vi "ConfigureTarget.vi"(8 "error in (no error)":errorcluster, 10 "TargetRate":dbl, 11 "Target Reference in":refnum<k24>) -> (0 "error out":errorcluster, 3 "Target Reference out":refnum<k24>)   [LabVIEW 2015, in "VeriStandTestUtilities.lvlib"]
uses:
  VeriStandTestUtilities.lvlib
  NationalInstruments.VeriStand.SystemDefinitionAPI
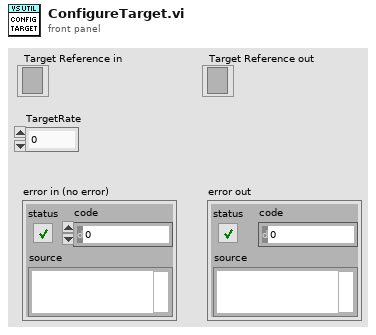
[diagram p1: front panel]
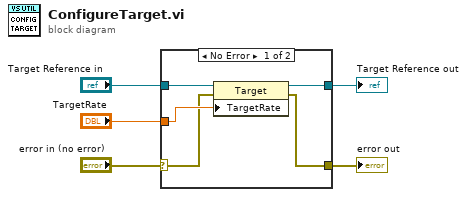
[diagram p0: block diagram]
diagram:
  n1 = case shown="No Error" "error in (no error)" {
    selector: "error in (no error)" -> [w6 w12]
    tunnel: [w10 w12] -> w5
    tunnel: [w9 w11] -> w4
    tunnel: "Target Reference in" -> [w8 w11]
    tunnel: "TargetRate" -> [w7 _]
    frame No Error {
      n2 = property class="Target"(reference=w8, error in=w6, "TargetRate"=w7) -> (reference out=w9:refnum<k24>, error out=w10:errorcluster)
    }
    frame Error {
    }
  }
  "error out" <- w5
  "Target Reference out" <- w4
